vi "BoxExecuteTuneShooter.vi"(8 "error in (no error)":errorcluster) -> (0 "error out":errorcluster)   [LabVIEW 2023]
uses:
  <vilib>/Rock Robotics/WPI/ThirdParty/JAS_Junk/TrajLib/TypeDef/PID_ERROR_TOLERANCE.ctl
  <vilib>/Rock Robotics/WPI/ThirdParty/JAS_Junk/TrajLib/VI/BoolCmd_Recv_Internal.vi
  <vilib>/Rock Robotics/WPI/ThirdParty/JAS_Junk/TrajLib/PIDController_AtSetpoint.vi
  <vilib>/Rock Robotics/WPI/ThirdParty/JAS_Junk/TrajLib/PIDController_SetPIDF.vi
  <vilib>/Rock Robotics/WPI/ThirdParty/JAS_Junk/TrajLib/PIDController_SetDerivativeFilter.vi
  <vilib>/Rock Robotics/WPI/ThirdParty/JAS_Junk/TrajLib/PIDController_SetIntegratorRange.vi
  <vilib>/Rock Robotics/WPI/ThirdParty/JAS_Junk/TrajLib/PIDController_SetTolerancePandV.vi
  <vilib>/Rock Robotics/WPI/ThirdParty/JAS_Junk/TrajLib/PIDController_DisableContinousInput.vi
  <vilib>/Rock Robotics/WPI/ThirdParty/JAS_Junk/TrajLib/PIDController_EnableContinousInput.vi
  <vilib>/Rock Robotics/WPI/ThirdParty/JAS_Junk/TrajLib/PIDController_Reset.vi
  <vilib>/Rock Robotics/WPI/ThirdParty/JAS_Junk/TrajLib/PIDController_New.vi
  <vilib>/Rock Robotics/WPI/ThirdParty/JAS_Junk/TrajLib/PIDController_SetOutputLimits.vi
  <vilib>/Rock Robotics/WPI/ThirdParty/JAS_Junk/TrajLib/SimpleMotorFF_Calculate.vi
  <vilib>/Rock Robotics/WPI/ThirdParty/JAS_Junk/TrajLib/LinearFilter_LowPassBW1.vi
  <vilib>/Rock Robotics/WPI/ThirdParty/JAS_Junk/TrajLib/LinearFilter_ResetToValue.vi
  <vilib>/Rock Robotics/WPI/ThirdParty/JAS_Junk/TrajLib/LinearFilter_Calculate.vi
  <vilib>/Rock Robotics/WPI/ThirdParty/JAS_Junk/TrajLib/SlewRateLimiter_New.vi
  <vilib>/Rock Robotics/WPI/ThirdParty/JAS_Junk/TrajLib/SlewRateLimiter_Reset.vi
  <vilib>/Rock Robotics/WPI/ThirdParty/JAS_Junk/TrajLib/SlewRateLimiter_Calculate.vi
  <vilib>/Rock Robotics/WPI/ThirdParty/JAS_Junk/TrajLib/SlewRateLimiter_SetRate.vi
  <vilib>/Rock Robotics/WPI/ThirdParty/JAS_Junk/TrajLib/VI/BoolCmd_ObtainQueue.vi
  <vilib>/Rock Robotics/WPI/ThirdParty/JAS_Junk/TrajLib/PIDController_NewPeriod.vi
  <vilib>/Rock Robotics/WPI/ThirdParty/JAS_Junk/TrajLib/LinearFilter_New.vi
  <vilib>/Rock Robotics/WPI/ThirdParty/JAS_Junk/TrajLib/Util_GetTime.vi
  <vilib>/Rock Robotics/SystemInterfaces/NetworkCommunication/NetComm_UsageReport_report.vi
  <vilib>/Rock Robotics/WPI/ThirdParty/JAS_Junk/TrajLib/VI/Util_GetTime_U32.vi
  <vilib>/Rock Robotics/Network Tables/NT Write Boolean.vi
  <vilib>/Rock Robotics/Network Tables/NT Write Number.vi
  <vilib>/Utility/semaphor.llb/Obtain Semaphore Reference.vi
  <vilib>/Rock Robotics/WPI/ThirdParty/JAS_Junk/TrajLib/Timer_Reset.vi
  <vilib>/Rock Robotics/WPI/ThirdParty/JAS_Junk/TrajLib/Timer_Start.vi
  <vilib>/Rock Robotics/WPI/ThirdParty/JAS_Junk/TrajLib/Timer_Stop.vi
  <vilib>/Rock Robotics/WPI/ThirdParty/JAS_Junk/TrajLib/LinearFilter_MovingAverage.vi
  <vilib>/Rock Robotics/WPI/ThirdParty/JAS_Junk/TrajLib/Globals/Util_LibraryGlobals.vi
  <vilib>/Rock Robotics/WPI/ThirdParty/JAS_Junk/TrajLib/LinearFilter_LowPassBW2.vi
  <vilib>/Rock Robotics/WPI/ThirdParty/JAS_Junk/TrajLib/LinearFilter_HighPassBW1.vi
  <vilib>/Rock Robotics/WPI/ThirdParty/JAS_Junk/TrajLib/LinearFilter_HighPassBW2.vi
  <vilib>/Rock Robotics/SystemInterfaces/Utilities/FPGA_UtilitiesRead LocalTime.vi
  <vilib>/Rock Robotics/WPI/ThirdParty/JAS_Junk/TrajLib/VI/Util_GetTime_U64.vi
  <vilib>/Rock Robotics/WPI/ThirdParty/JAS_Junk/TrajLib/PIDController_AdvCalculate_FF_Sp_Pv.vi
  <vilib>/Rock Robotics/WPI/ThirdParty/JAS_Junk/TrajLib/Trajectory_Library.lvlib
  <vilib>/Rock Robotics/Network Tables/NT Read Number.vi
  <vilib>/Rock Robotics/WPI/Joystick/XBox Buttons Indexer.ctl
panel:
  # "Click here to set min"
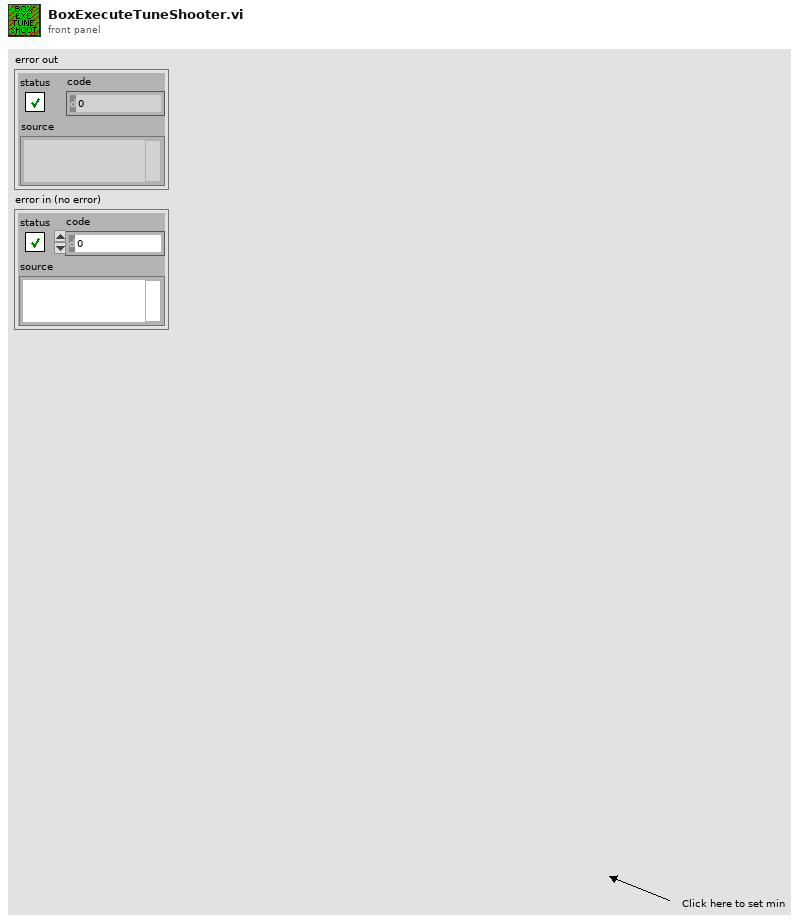
[diagram p1: front panel]
types:
  T1 = typedef "XBox Buttons Indexer.ctl" = enum16{"A", "B", "X", "Y", "Left Bumper", "Right Bumper", "Back", "Start", "Left Joystick", "Right Joystick"}
  T2 = enum16{"Ziegler Nicols - Fast", "Ziegler Nicols - Normal", "Ziegler Nicols - Slow", "CHR regulator - 0% overshoot", "CHR regulator - 20% overshoot", "CHR servo - 0 % overshoot", "CHR servo - 20% overshoot"}
  T3 = enum16{"Moving Average", "Low Pass 1st Order Butterworth", "Low Pass 2nd Order Butterworth", "High Pass 1st Order Butterworth", "High Pass 2nd Order Butterworth"}
  T4 = typedef "Trajectory_Library.lvlib/PID_ERROR_TOLERANCE.ctl" = cluster{"PositionTolerance":dbl, "VelocityTolerance":dbl}
  T5 = typedef "WPI_JoystickDevRef.ctl" = cluster{"Device":T6}
  T6 = typedef "WPI_JoystickDeviceEnum.ctl" = enum16{"USB 0", "USB 1", "USB 2", "USB 3", "USB 4", "USB 5"}
  T7 = typedef "WPI_MotorControlDeviceRef.ctl" = cluster{"DeviceStatus":errorcluster, "Type":T8, "PWM":cluster{"PWM Channel":T9, "DeadBand":T10}, "CAN":cluster{"Device Number":u8, "SetOutput VI Ref":variant, "GetOutput VI Ref":variant, "Enable VI Ref":variant, "Disable VI Ref":variant, "Data":variant}, "Invert":bool, "DIO PWM":cluster{"PWM \"Enable\" Channel":T9, "DIOChannel":T11, "PWM Rate":dbl}}
  T8 = typedef "WPI_MotorControlType.ctl" = enum16{"PWM", "CAN", "DIO PWM"}
  T9 = typedef "FPGA_DIOPWMChannel.ctl" = enum8{"PWM 0", "PWM 1", "PWM 2", "PWM 3", "PWM 4", "PWM 5", "PWM 6", "PWM 7", "PWM 8", "PWM 9", "PWM MXP 0", "PWM MXP 1", "PWM MXP 2", "PWM MXP 3", "PWM MXP 4", "PWM MXP 5", "PWM MXP 6", "PWM MXP 7", "PWM MXP 8", "PWM MXP 9", "Invalid"}
  T10 = typedef "WPI_PWMDeadband.ctl" = cluster{"Name":string, "maxPositivePwm":i32, "minPositivePwm":i32, "centerPwm":i32, "maxNegativePwm":i32, "minNegativePwm":i32, "angularRange":u16}
  T11 = typedef "FPGA_DIOChannel.ctl" = enum8{"DIO 0", "DIO 1", "DIO 2", "DIO 3", "DIO 4", "DIO 5", "DIO 6", "DIO 7", "DIO 8", "DIO 9", "DIO MXP 0", "DIO MXP 1", "DIO MXP 2", "DIO MXP 3", "DIO MXP 4", "DIO MXP 5", "DIO MXP 6", "DIO MXP 7", "DIO MXP 8", "DIO MXP 9", "DIO MXP 10", "DIO MXP 11", "DIO MXP 12", "DIO MXP 13", "DIO MXP 14", "DIO MXP 15", "SPI Port CS1", "SPI Port CS2", "SPI Port CS3", "SPI Port MISO", "SPI Port MOSI", "Invalid"}
  T12 = typedef "Trajectory_Library.lvlib/SIMPLE_MOTOR_FF.ctl" = cluster{"Ks":dbl, "Kv":dbl, "Ka":dbl, "KnInv":dbl}
  T13 = typedef "Trajectory_Library.lvlib/PID_ADV_TUNING.ctl" = cluster{"Kf":dbl, "Kp":dbl, "Ki":dbl, "Kd":dbl, "MaximumIntegral":dbl, "MinimumIntegral":dbl, "Filter Derivative":bool}
  T14 = typedef "Trajectory_Library.lvlib/PID_ADV_LIMITS.ctl" = cluster{"MaxInput":dbl, "MinInput":dbl, "Continuous":bool, "MaxOutput":dbl, "MinOutput":dbl}
  T15 = cluster{"Controller Constant Type":enum16{"Ziegler Nicols - Fast", "Ziegler Nicols - Normal", "Ziegler Nicols - Slow", "CHR regulator - 0% overshoot", "CHR regulator - 20% overshoot", "CHR servo - 0 % overshoot", "CHR servo - 20% overshoot"}, "Type of Controller":enum16{"P", "PI", "PID"}, "CO Offset":dbl, "Kn":dbl, "Tuning Tolerance":dbl, "Plant Tolerance":dbl, "Newest Avg Time ":i32, "Long Ave Time":i32}
  T16 = cluster{"Plant Gain (K)":dbl, "Time Constant (T)":dbl, "Dead Time (L)":dbl, "stimulus operating point":dbl, "response operating point":dbl}
  T17 = cluster{"proportional gain (Kp)":dbl, "integral time (Ki / Sec)":dbl, "derivative time (Kd /Sec)":dbl}
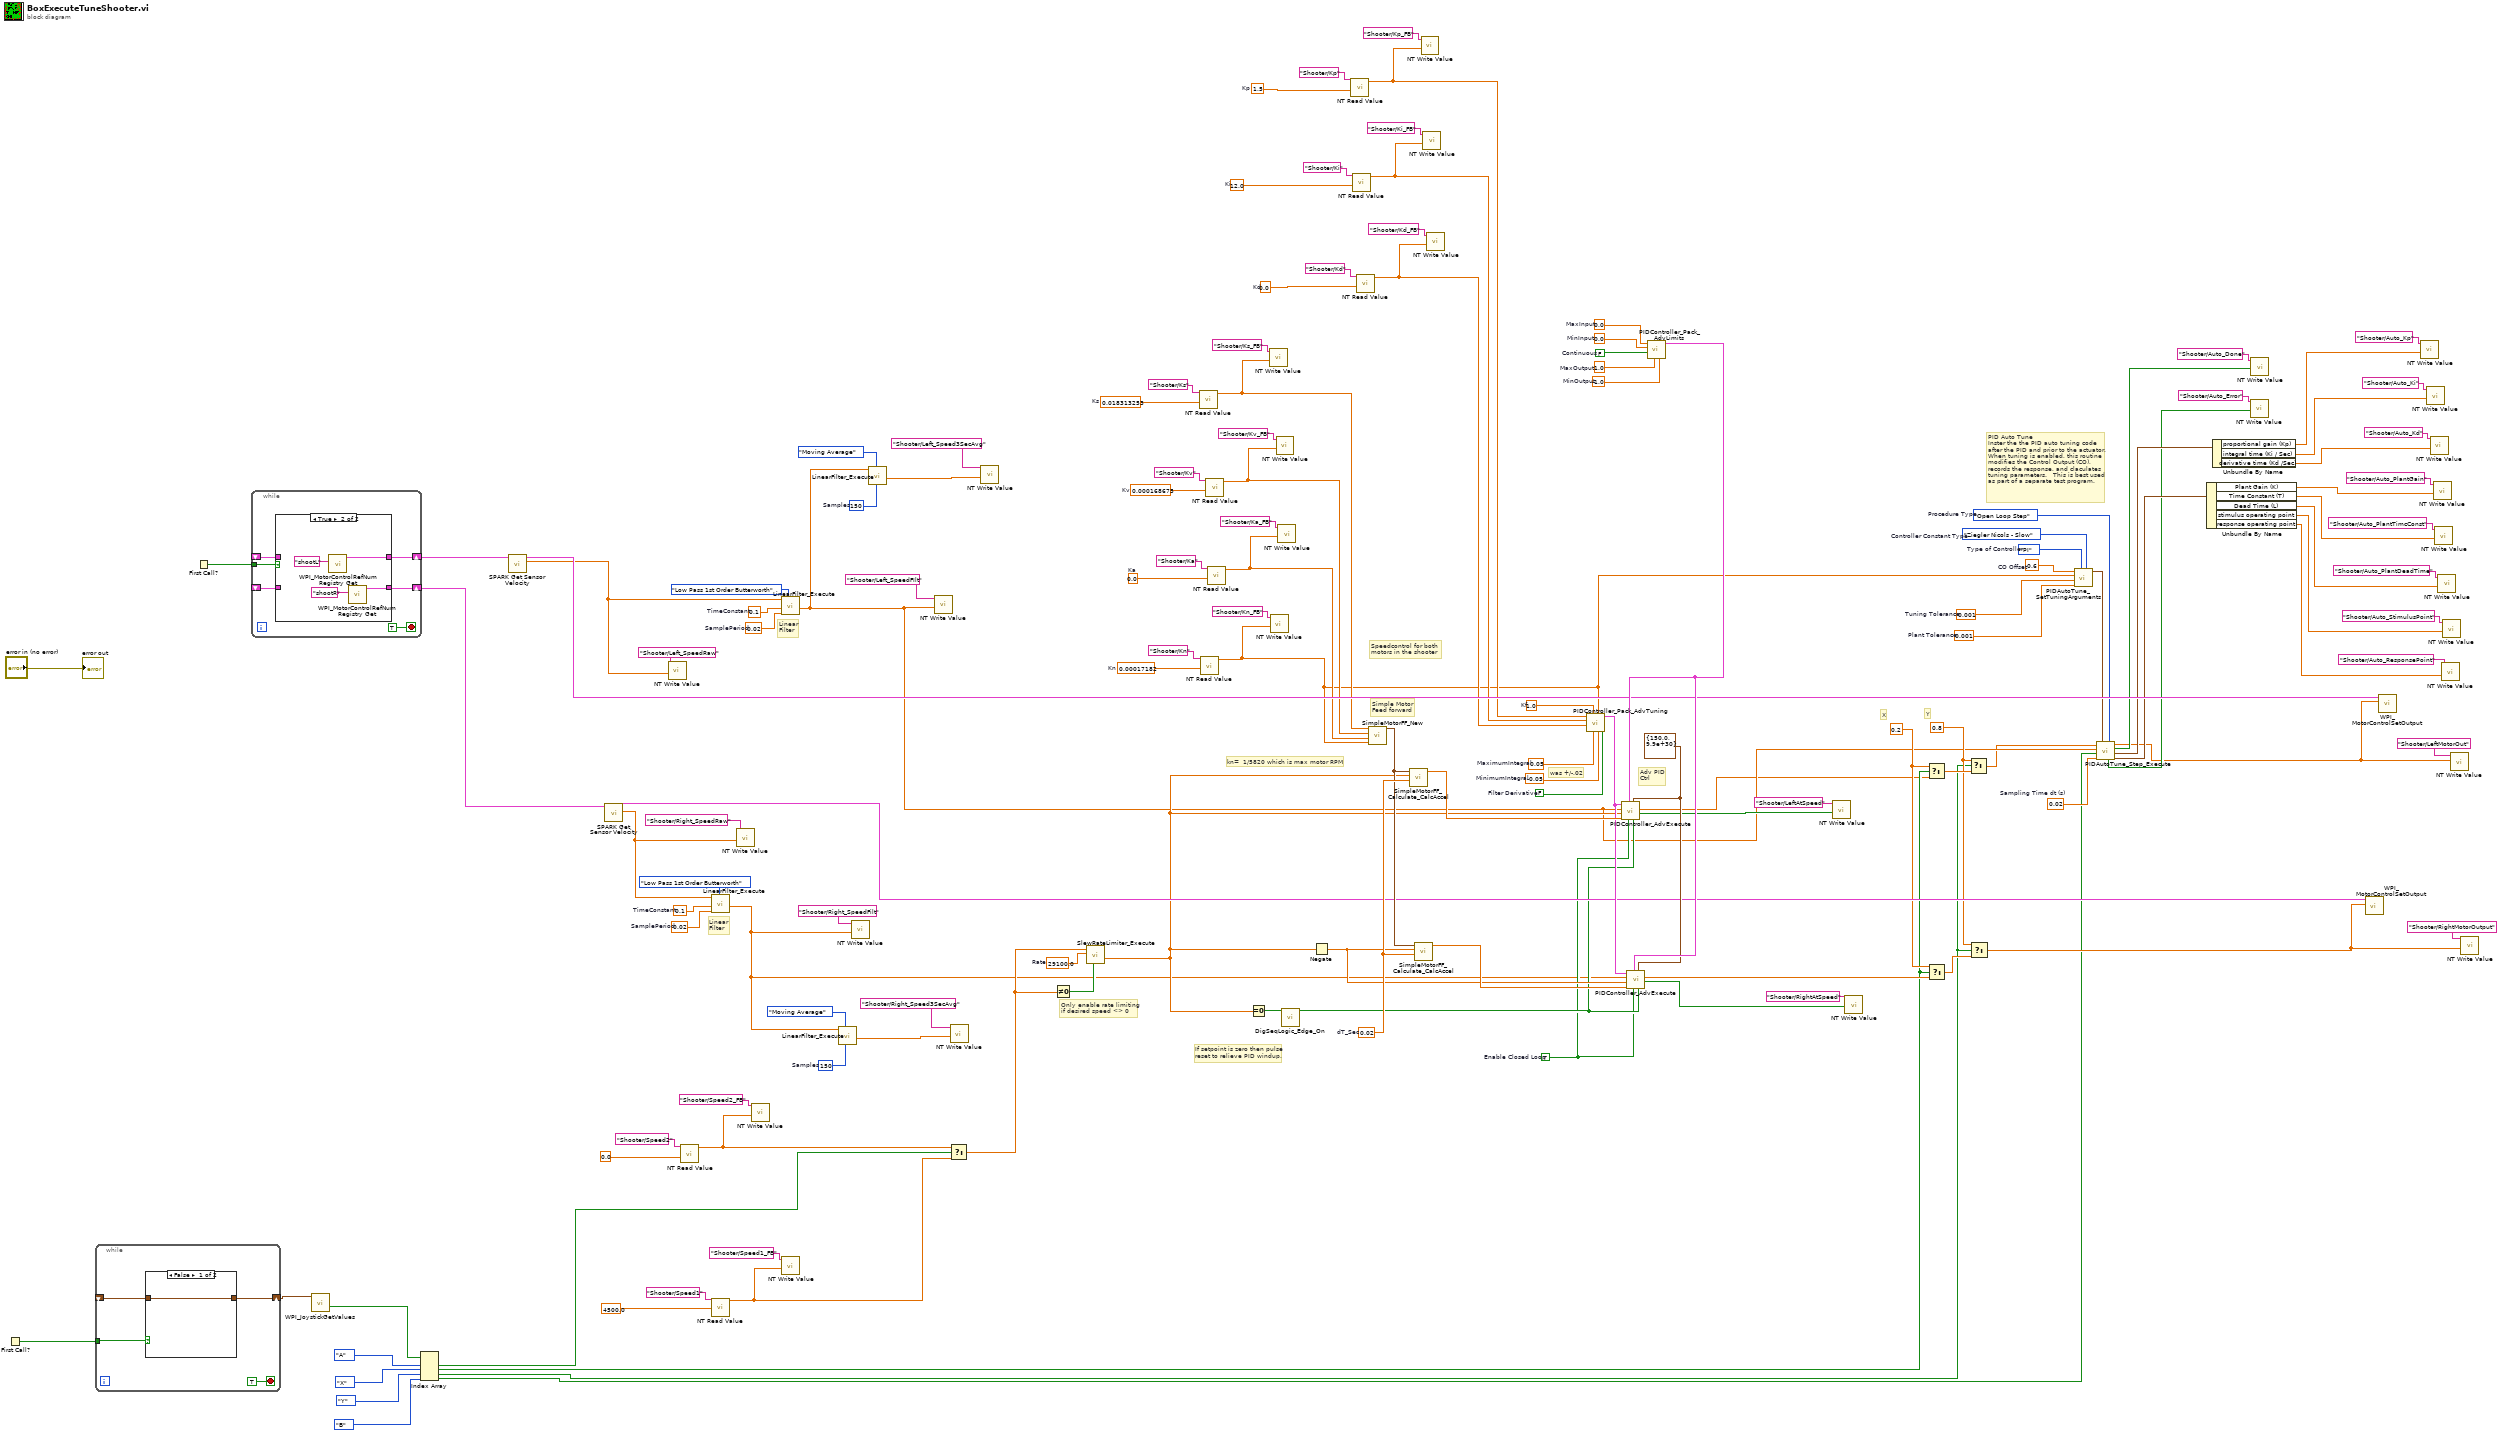
[diagram p0: block diagram]
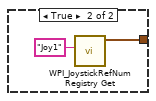
[diagram p2: hidden frame]
diagram:
  w29 = 0.001  # Plant Tolerance
  w30 = 0.001  # Tuning Tolerance
  w37 = 0.02  # Sampling Time dt (s)
  w36 = 0.6  # CO Offset
  w35 = enum16{"P", "PI", "PID"}."PI"  # Type of Controller
  w34 = T2."Ziegler Nicols - Slow"  # Controller Constant Type
  w33 = enum16{"Open Loop Step", "Closed Loop Step"}."Open Loop Step"  # Procedure Type
  w40 = 0.8
  w41 = 0.2
  w52 = 150  # Samples
  w57 = 150  # Samples
  w103 = 29100.0  # Rate
  w118 = 0.02  # SamplePeriod
  w117 = 0.1  # TimeConstant
  w123 = 0.02  # SamplePeriod
  w122 = 0.1  # TimeConstant
  w101 = TRUE  # Enable Closed Loop
  w126 = T4 {"PositionTolerance"=150.0, "VelocityTolerance"=9.9e+30} ("PID Error Tolerance")
  w84 = 0.00017182  # Kn
  w98 = 0.018313253  # Ks
  w92 = 0.000168675  # Kv
  w88 = 0.0  # Ka
  w74 = 1.5  # Kp
  w75 = 12.0  # Ki
  w77 = 0.0  # Kd
  w134 = 1.0  # Kf
  w133 = 0.05  # MaximumIntegral
  w132 = -0.05  # MinimumIntegral
  w131 = FALSE  # Filter Derivative
  w138 = 0.0  # MinInput
  w137 = FALSE  # Continuous
  w136 = 1.0  # MaxOutput
  w135 = -1.0  # MinOutput
  w139 = 0.0  # MaxInput
  w130 = 0.02  # dT_Sec
  # "PID Auto Tune\nInster the the PID auto tuning code\nafter the PID and prior to the actuator.\nWhen tuning is enabled, this routine\nmodifies the Control Output (CO), \nrecords the response, and claculates\ntuning parameters.   This is best used\nas part of a separate test program."
  # "Y"
  # "X"
  # "was +/-.02"
  # "If setpoint is zero then pulse\nreset to relieve PID windup."
  # "Only enable rate limiting\nif desired speed <> 0"
  # "Linear\nFilter"
  # "Linear\nFilter"
  # "Speedcontrol for both \nmotors in the shooter"
  # "Simple Motor\nFeed forward"
  # "Adv PID\nCtrl"
  # "kn=  1/5820 which is max motor RPM"
  n1 = First Call?() -> (First Call?: T/F=w62:bool)
  n2 = while {
    tunnel: w62 -> [w148]
    shift-right: [w146] -> w61
    shift-left: _ -> [w145]
    stop <- TRUE stop-if-true
    n3 = case shown="False" w148 {
      tunnel: [w149 w150] -> w146
      tunnel: w145 -> [w149 _]
      frame False {
      }
      frame True {
        n4 = call <vilib>:"WPI_JoystickRefNum Registry Get.vi"("refnum name"="Joy1") -> ("JoystickDevRef"=w150:T5)  [unwired: 9 in, 1 out]
      }
    }
  }
  n5 = First Call?() -> (First Call?: T/F=w100:bool)
  n6 = while {
    tunnel: w100 -> [w155]
    shift-right: [w157] -> w143
    shift-left: _ -> [w153]
    shift-right: [w156] -> w142
    shift-left: _ -> [w152]
    stop <- TRUE stop-if-true
    n7 = case shown="True" w155 {
      tunnel: [w159 w161] -> w157
      tunnel: [w158 w160] -> w156
      tunnel: w153 -> [w159 _]
      tunnel: w152 -> [w158 _]
      frame False {
      }
      frame True {
        n8 = call <vilib>:"WPI_MotorControlRefNum Registry Get.vi"("refnum name"="shootL") -> ("MotorControlDevRef"=w161:T7)  [unwired: 9 in, 1 out]
        n9 = call <vilib>:"WPI_MotorControlRefNum Registry Get.vi"("refnum name"="shootR") -> ("MotorControlDevRef"=w160:T7)  [unwired: 9 in, 1 out]
      }
    }
  }
  n10 = call <vilib>:"WPI_JoystickGetValues.vi"("JoystickDevRef"=w61) -> ("Buttons"=w60:bool[])  [unwired: 6 in, 4 out]
  n11 = Index Array(array=w60, index #1=XBox_Buttons_Indexer."A" ("XBox Buttons"), index #2=XBox_Buttons_Indexer."X" ("XBox Buttons"), index #3=XBox_Buttons_Indexer."Y" ("XBox Buttons"), index #4=XBox_Buttons_Indexer."B" ("XBox Buttons")) -> (element #1=w58:bool, element #2=w39:bool, element #3=w38:bool, element #4=w4:bool)
  n12 = call <vilib>:"SPARK Get Sensor Velocity.vi"("MotorControlDevRef in"=w143) -> ("Sensor Velocity"=w55:dbl, "MotorControlDevRef out"=w119:T7)  [unwired: 7 in, 2 out]
  n13 = call <vilib>:"SPARK Get Sensor Velocity.vi"("MotorControlDevRef in"=w142) -> ("Sensor Velocity"=w120:dbl, "MotorControlDevRef out"=w110:T7)  [unwired: 7 in, 2 out]
  n14 = call-poly <vilib>:"NT Write Value.vi"("value"=w55, "name"="Shooter/Left_SpeedRaw") -> ()  [unwired: 9 in, 1 out]
  n15 = call-poly <vilib>:"NT Read Value.vi"("default value"=0.0, "name"="Shooter/Speed2") -> ("value"=w66:dbl)  [unwired: 7 in, 2 out]
  n16 = call <vilib>:"LinearFilter_Execute.vi"("Filter Type"=T3."Low Pass 1st Order Butterworth", "SamplePeriod"=w123, "TimeConstant"=w122, "Input"=w120) -> ("Output"=w48:dbl)  [unwired: 6 in, 1 out]
  n17 = call-poly <vilib>:"NT Read Value.vi"("default value"=4500.0, "name"="Shooter/Speed1") -> ("value"=w65:dbl)  [unwired: 7 in, 2 out]
  n18 = call-poly <vilib>:"NT Write Value.vi"("value"=w120, "name"="Shooter/Right_SpeedRaw") -> ()  [unwired: 9 in, 1 out]
  n19 = call-poly <vilib>:"NT Write Value.vi"("value"=w66, "name"="Shooter/Speed2_FB") -> ()  [unwired: 9 in, 1 out]
  n20 = call <vilib>:"LinearFilter_Execute.vi"("Filter Type"=T3."Low Pass 1st Order Butterworth", "SamplePeriod"=w118, "TimeConstant"=w117, "Input"=w55) -> ("Output"=w5:dbl)  [unwired: 6 in, 1 out]
  n21 = call-poly <vilib>:"NT Write Value.vi"("value"=w65, "name"="Shooter/Speed1_FB") -> ()  [unwired: 9 in, 1 out]
  n22 = call <vilib>:"LinearFilter_Execute.vi"("Samples"=w52, "Filter Type"=T3."Moving Average", "Input"=w48) -> ("Output"=w49:dbl)  [unwired: 7 in, 1 out]
  n23 = call-poly <vilib>:"NT Write Value.vi"("value"=w48, "name"="Shooter/Right_SpeedFilt") -> ()  [unwired: 9 in, 1 out]
  n24 = call <vilib>:"LinearFilter_Execute.vi"("Samples"=w57, "Filter Type"=T3."Moving Average", "Input"=w5) -> ("Output"=w53:dbl)  [unwired: 7 in, 1 out]
  n25 = call-poly <vilib>:"NT Write Value.vi"("value"=w5, "name"="Shooter/Left_SpeedFIlt") -> ()  [unwired: 9 in, 1 out]
  n26 = call-poly <vilib>:"NT Write Value.vi"("value"=w49, "name"="Shooter/Right_Speed3SecAvg") -> ()  [unwired: 9 in, 1 out]
  n27 = Select(t=w66, s=w58, f=w65) -> (s? t:f=w71:dbl)
  n28 = call-poly <vilib>:"NT Write Value.vi"("value"=w53, "name"="Shooter/Left_Speed3SecAvg") -> ()  [unwired: 9 in, 1 out]
  n29 = Not Equal To 0?(x=w71) -> (x != 0?=w102:bool)
  n30 = call <vilib>:"SlewRateLimiter_Execute.vi"("Enable"=w102, "PositiveRate"=w103, "Input"=w71) -> ("Output"=w99:dbl)  [unwired: 7 in, 1 out]
  n31 = call-poly <vilib>:"NT Read Value.vi"("default value"=w98, "name"="Shooter/Ks") -> ("value"=w95:dbl)  [unwired: 7 in, 2 out]
  n32 = call-poly <vilib>:"NT Read Value.vi"("default value"=w84, "name"="Shooter/Kn") -> ("value"=w31:dbl)  [unwired: 7 in, 2 out]
  n33 = call-poly <vilib>:"NT Read Value.vi"("default value"=w92, "name"="Shooter/Kv") -> ("value"=w91:dbl)  [unwired: 7 in, 2 out]
  n34 = call-poly <vilib>:"NT Read Value.vi"("default value"=w88, "name"="Shooter/Ka") -> ("value"=w87:dbl)  [unwired: 7 in, 2 out]
  n35 = Equal To 0?(x=w99) -> (x = 0?=w105:bool)
  n36 = call-poly <vilib>:"NT Write Value.vi"("value"=w95, "name"="Shooter/Ks_FB") -> ()  [unwired: 9 in, 1 out]
  n37 = call-poly <vilib>:"NT Write Value.vi"("value"=w31, "name"="Shooter/Kn_FB") -> ()  [unwired: 9 in, 1 out]
  n38 = call-poly <vilib>:"NT Write Value.vi"("value"=w91, "name"="Shooter/Kv_FB") -> ()  [unwired: 9 in, 1 out]
  n39 = call-poly <vilib>:"NT Write Value.vi"("value"=w87, "name"="Shooter/Ka_FB") -> ()  [unwired: 9 in, 1 out]
  n40 = call <vilib>:"DigSeqLogic_Edge_On.vi"("Input"=w105) -> ("On Edge"=w104:bool)  [unwired: 10 in]
  n41 = Negate(x=w99) -> (-x=w124:dbl)
  n42 = call-poly <vilib>:"NT Read Value.vi"("default value"=w74, "name"="Shooter/Kp") -> ("value"=w72:dbl)  [unwired: 7 in, 2 out]
  n43 = call-poly <vilib>:"NT Read Value.vi"("default value"=w75, "name"="Shooter/Ki") -> ("value"=w73:dbl)  [unwired: 7 in, 2 out]
  n44 = call-poly <vilib>:"NT Read Value.vi"("default value"=w77, "name"="Shooter/Kd") -> ("value"=w76:dbl)  [unwired: 7 in, 2 out]
  n45 = call <vilib>:"SimpleMotorFF_New.vi"("Kn"=w31, "Ka"=w87, "Kv"=w91, "Ks"=w95) -> ("SIMPLE_MOTOR_FF"=w129:T12)  [unwired: 7 in]
  n46 = call <vilib>:"SimpleMotorFF_Calculate_CalcAccel.vi"("dT_Sec"=w130, "VelSp"=w99, "SIMPLE_MOTOR_FF"=w129) -> ("FeedForward"=w140:dbl)  [unwired: 8 in]
  n47 = call <vilib>:"SimpleMotorFF_Calculate_CalcAccel.vi"("dT_Sec"=w130, "VelSp"=w124, "SIMPLE_MOTOR_FF"=w129) -> ("FeedForward"=w125:dbl)  [unwired: 8 in]
  n48 = call-poly <vilib>:"NT Write Value.vi"("value"=w72, "name"="Shooter/Kp_FB") -> ()  [unwired: 9 in, 1 out]
  n49 = call-poly <vilib>:"NT Write Value.vi"("value"=w73, "name"="Shooter/Ki_FB") -> ()  [unwired: 9 in, 1 out]
  n50 = call-poly <vilib>:"NT Write Value.vi"("value"=w76, "name"="Shooter/Kd_FB") -> ()  [unwired: 9 in, 1 out]
  n51 = call <vilib>:"PIDController_Pack_AdvTuning.vi"("Filter Derivative"=w131, "MinimumIntegral"=w132, "Kn"=w31, "MaximumIntegral"=w133, "Kf"=w134, "Kd"=w76, "Ki"=w73, "Kp"=w72) -> ("Adv PID Tuning"=w128:T13)  [unwired: 3 in]
  n52 = call <vilib>:"PIDController_Pack_AdvLimits.vi"("MinOutput"=w135, "MaxOutput"=w136, "Continuous"=w137, "MinInput"=w138, "MaxInput"=w139) -> ("Adv PID Limits"=w127:T14)  [unwired: 6 in]
  n53 = call <vilib>:"PIDController_AdvExecute.vi"("Reset"=w104, "PID Error Tolerance"=w126, "Auto"=w101, "Adv PID Limits"=w127, "FF-FeedForward"=w140, "SP-SetPoint"=w99, "PV-Measurement"=w5, "Adv PID Tuning"=w128) -> ("AtSetpoint"=w114:bool, "CO-ControlOutput"=w1:dbl)  [unwired: 1 in, 1 out]
  n54 = call <vilib>:"PIDController_AdvExecute.vi"("Reset"=w104, "PID Error Tolerance"=w126, "Auto"=w101, "Adv PID Limits"=w127, "FF-FeedForward"=w125, "SP-SetPoint"=w124, "PV-Measurement"=w48, "Adv PID Tuning"=w128) -> ("AtSetpoint"=w115:bool, "CO-ControlOutput"=w42:dbl)  [unwired: 1 in, 1 out]
  n55 = call-poly <vilib>:"NT Write Value.vi"("value"=w114, "name"="Shooter/LeftAtSpeed") -> ()  [unwired: 9 in, 1 out]
  n56 = call-poly <vilib>:"NT Write Value.vi"("value"=w115, "name"="Shooter/RightAtSpeed") -> ()  [unwired: 9 in, 1 out]
  n57 = Select(t=w41, s=w39, f=w1) -> (s? t:f=w45:dbl)
  n58 = Select(t=w41, s=w39, f=w42) -> (s? t:f=w44:dbl)
  n59 = Select(t=w40, s=w38, f=w45) -> (s? t:f=w2:dbl)
  n60 = Select(t=w40, s=w38, f=w44) -> (s? t:f=w43:dbl)
  n61 = call <vilib>:"PIDAutoTune_SetTuningArguments.vi"("Controller Constant Type"=w34, "Type of Controller"=w35, "Plant Tolerance"=w29, "Tuning Tolerance"=w30, "Kn"=w31, "CO Offset"=w36) -> ("Configuration Parameters"=w32:T15)  [unwired: 5 in]
  n62 = call <vilib>:"PIDAutoTune_Step_Execute.vi"("Procedure Type"=w33, "Configuration Parameters"=w32, "Sampling Time dt (s)"=w37, "Tune"=w4, "Measurement  (PV)"=w5, "Control Output (Co)"=w2) -> ("Plant and Test Data"=w25:T16, "New Tuning Parameters"=w26:T17, "Tuning Done"=w27:bool, "Adj CO"=w3:dbl, "Error Occured"=w23:bool)  [unwired: 1 out]
  n63 = Unbundle By Name(w25) -> ("Plant Gain (K)"=w11:dbl, "Time Constant (T)"=w10:dbl, "Dead Time (L)"=w9:dbl, "stimulus operating point"=w8:dbl, "response operating point"=w7:dbl)
  n64 = Unbundle By Name(w26) -> ("proportional gain (Kp)"=w14:dbl, "integral time (Ki / Sec)"=w13:dbl, "derivative time (Kd /Sec)"=w12:dbl)
  n65 = call-poly <vilib>:"NT Write Value.vi"("value"=w23, "name"="Shooter/Auto_Error") -> ()  [unwired: 9 in, 1 out]
  n66 = call-poly <vilib>:"NT Write Value.vi"("value"=w27, "name"="Shooter/Auto_Done") -> ()  [unwired: 9 in, 1 out]
  n67 = call <vilib>:"WPI_MotorControlSetOutput.vi"("Output"=w43, "MotorControlDevRef"=w110) -> ()  [unwired: 7 in, 3 out]
  n68 = call <vilib>:"WPI_MotorControlSetOutput.vi"("Output"=w3, "MotorControlDevRef"=w119) -> ()  [unwired: 7 in, 3 out]
  n69 = call-poly <vilib>:"NT Write Value.vi"("value"=w14, "name"="Shooter/Auto_Kp") -> ()  [unwired: 9 in, 1 out]
  n70 = call-poly <vilib>:"NT Write Value.vi"("value"=w13, "name"="Shooter/Auto_Ki") -> ()  [unwired: 9 in, 1 out]
  n71 = call-poly <vilib>:"NT Write Value.vi"("value"=w12, "name"="Shooter/Auto_Kd") -> ()  [unwired: 9 in, 1 out]
  n72 = call-poly <vilib>:"NT Write Value.vi"("value"=w11, "name"="Shooter/Auto_PlantGain") -> ()  [unwired: 9 in, 1 out]
  n73 = call-poly <vilib>:"NT Write Value.vi"("value"=w10, "name"="Shooter/Auto_PlantTimcConst") -> ()  [unwired: 9 in, 1 out]
  n74 = call-poly <vilib>:"NT Write Value.vi"("value"=w9, "name"="Shooter/Auto_PlantDeadTime") -> ()  [unwired: 9 in, 1 out]
  n75 = call-poly <vilib>:"NT Write Value.vi"("value"=w7, "name"="Shooter/Auto_ResponsePoint") -> ()  [unwired: 9 in, 1 out]
  n76 = call-poly <vilib>:"NT Write Value.vi"("value"=w8, "name"="Shooter/Auto_StimulusPoint") -> ()  [unwired: 9 in, 1 out]
  n77 = call-poly <vilib>:"NT Write Value.vi"("value"=w3, "name"="Shooter/LeftMotorOut") -> ()  [unwired: 9 in, 1 out]
  n78 = call-poly <vilib>:"NT Write Value.vi"("value"=w43, "name"="Shooter/RightMotorOutput") -> ()  [unwired: 9 in, 1 out]
  "error out" <- "error in (no error)"
